vi "Exp Moments.vi"(9 "b":dbl=1.0, 10 "a":dbl) -> (0 "error":i32, 2 "variance":dbl=1.0, 3 "mean":dbl)   [LabVIEW 2020, in "NI_Gmath.lvlib"]
doc: "Returns the expected mean and variance of the random variate X, where X describes the selected distribution type. You must manually select the polymorphic instance to use."
uses:
  <vilib>/gmath/NI_Gmath.lvlib
  <vilib>/gmath/statdist.llb/st_error_code.ctl
panel:
  # "Exp Moments"
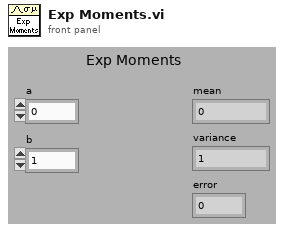
[diagram p1: front panel]
types:
  T1 = typedef "NI_Gmath.lvlib/st_error_code.ctl" = i32
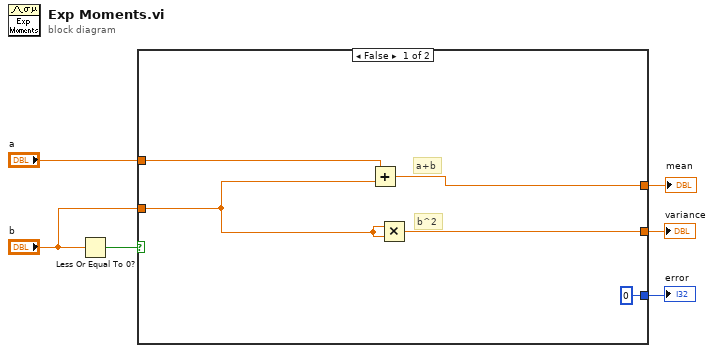
[diagram p0: block diagram]
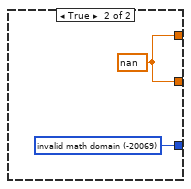
[diagram p2: hidden frame]
diagram:
  n1 = Less Or Equal To 0?(x="b") -> (x <= 0?=w3:bool)
  n2 = case shown="False" w3 {
    tunnel: "b" -> [w9 _]
    tunnel: [0 ("invalid math domain") w12] -> w6
    tunnel: [w7 w13] -> w5
    tunnel: "a" -> [w8 _]
    tunnel: [w10 w13] -> w1
    frame False {
      # "b^2"
      # "a+b"
      n3 = Add(x=w8, y=w9) -> (x+y=w7:dbl)
      n4 = Multiply(x=w9, y=w9) -> (x*y=w10:dbl)
    }
    frame True {
      w12 = T1 -20069 items=["invalid math domain"=-20069, "Fourier interpolation size m >= n"=-20070, "empty array"=-20003] ("stat interp error code")
      w13 = nan
    }
  }
  "mean" <- w5
  "error" <- w6
  "variance" <- w1
